vi "PH_IEEE1394Camera.reorder wanted Cam Attributes.vi"(2 "Name of Cam Attribute \"Video Mode\"":string, 3 "Wanted Attributes":T1(array[cluster])) -> (0 "redordered Wanted Attributes":T1(array[cluster]), 1 "Video Mode is going to be changed and at first array position":bool)   [LabVIEW 2014, in "PH_IEEE1394Camera.lvlib"]
uses:
  PH_IEEE1394Camera.lvlib
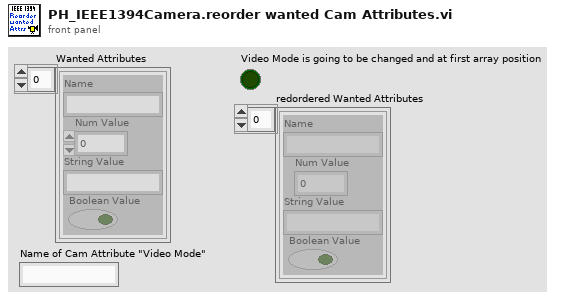
[diagram p1: front panel]
types:
  T1 = cluster{"Name":string, "Num Value":dbl, "String Value":string, "Boolean Value":bool}[]
  T2 = cluster{"Name":string, "Num Value":dbl, "String Value":string, "Boolean Value":bool}
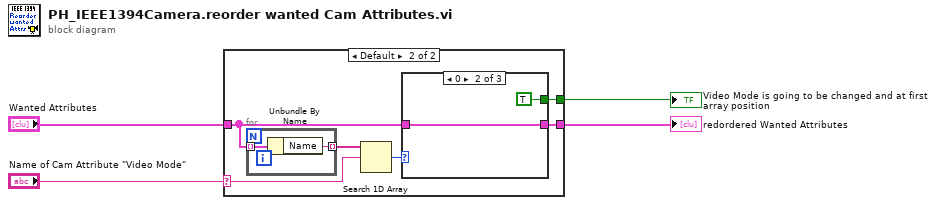
[diagram p0: block diagram]
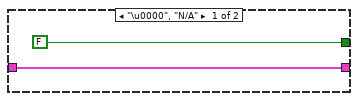
[diagram p2: hidden frame]
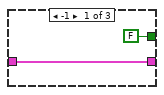
[diagram p3: hidden frame]
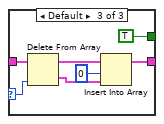
[diagram p4: hidden frame]
diagram:
  n1 = case shown="Default" "Name of Cam Attribute \"Video Mode\"" {
    selector: "Name of Cam Attribute \"Video Mode\"" -> [_ w9]
    tunnel: [w6 w12] -> w4
    tunnel: "Wanted Attributes" -> [w6 w10]
    tunnel: [FALSE ("Video Mode is going to be changed and moved to first array position") w11] -> w3
    frame "\u0000", "N/A" {
    }
    frame Default {
      n2 = for {
        tunnel: w10 -> [w25] mode=indexing
        tunnel: [w24] -> w8 mode=indexing
        n3 = Unbundle By Name(w25) -> ("Name"=w24:string)
      }
      n4 = Search 1D Array(1D array=w8, element=w9) -> (index of element=w7:i32)  [unwired: 1 in]
      n5 = case shown="0" w7 {
        selector: w7 -> [_ _ w17]
        tunnel: [w14 w16 w21] -> w12
        tunnel: [FALSE ("Video Mode is going to be changed and moved to first array position") TRUE ("Video Mode is going to be changed and moved to first array position") TRUE ("Video Mode is going to be changed and moved to first array position")] -> w11
        tunnel: w10 -> [w14 w16 w18]
        frame -1 {
        }
        frame 0 {
        }
        frame Default {
          n6 = Delete From Array(array=w18, index=w17) -> (deleted portion=w19:T2, array with subset deleted=w23:T1)  [unwired: 1 in]
          n7 = Insert Into Array(array=w23, index=0, new element=w19) -> (w21:T1)
        }
      }
    }
  }
  "redordered Wanted Attributes" <- w4
  "Video Mode is going to be changed and at first array position" <- w3
